vi "Error Checking Unpacker.vi"(8 "error in":errorcluster, 10 "packed i12s":i16[](array[numeric])=[0, 16, 32, 48, 64, 80, 96, 112, 2049, 2305, 2561, 2817, 3073, 3329, 3585, 3841, 24, 4121, 8218, 12315, 16412, 20509, 24606, 28703] format="%016b") -> (0 "error out":errorcluster)   [LabVIEW 2012]
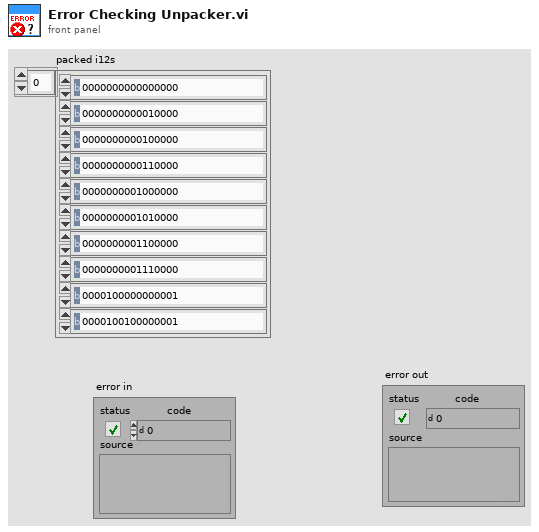
[diagram p1: front panel]
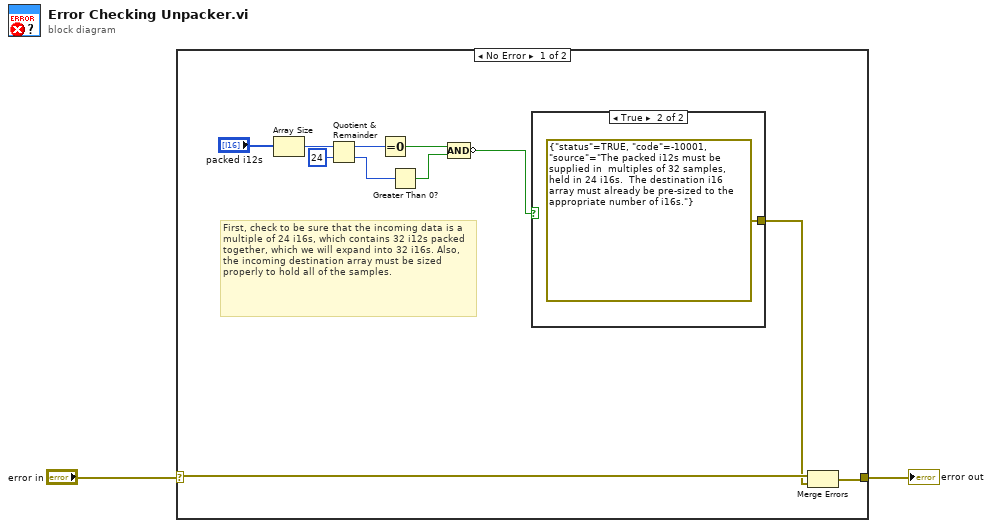
[diagram p0: block diagram]
diagram:
  n1 = case shown="No Error" "error in" {
    selector: "error in" -> [w5 w15]
    tunnel: [w6 w15] -> w1
    frame No Error {
      # "First, check to be sure that the incoming data is a multiple of 24 i16s, which contains 32 i12s packed together, which we will expand into 32 i16s. Also, the incoming destination array must be sized properly to hold all of the samples."
      n2 = Array Size(array="packed i12s") -> (size(s)=w8:i32)
      n3 = Quotient & Remainder(x=w8, y=24) -> (x-y*floor(x/y)=w13:i32, floor(x/y)=w7:i32)
      n4 = Equal To 0?(x=w13) -> (x = 0?=w11:bool)
      n5 = Greater Than 0?(x=w7) -> (x > 0?=w10:bool)
      n6 = Compound Arithmetic op=AND(w11, w10) -> (invert w3:bool)
      n7 = case shown="True" w3 {
        tunnel: [_ errorcluster {"status"=TRUE, "code"=-10001, "source"="The packed i12s must be supplied in  multiples of 32 samples, held in 24 i16s.  The destination i16 array must already be pre-sized to the appropriate number of i16s."} ("error IO")] -> w4
        frame False {
        }
        frame True {
        }
      }
      n8 = Merge Errors(w5, w4) -> (w6:errorcluster)
    }
    frame Error {
    }
  }
  "error out" <- w1
